vi "MM-TimeSpanText.vi"(4 "Timespan":dbl) -> (1 "TimeSpanText":string)   [LabVIEW 2020]
doc: "Show timespan in text format"
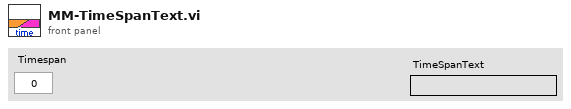
[diagram p1: front panel]
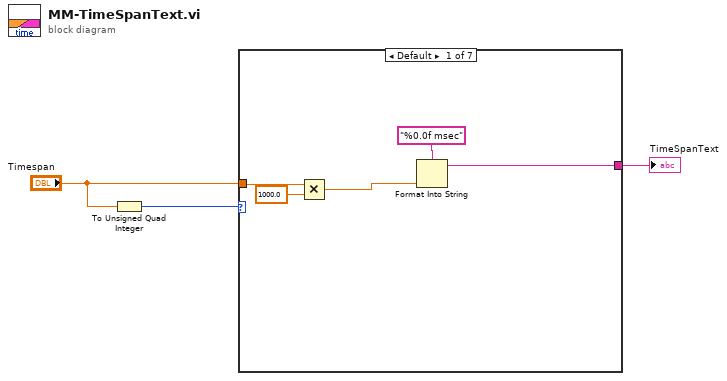
[diagram p0: block diagram]
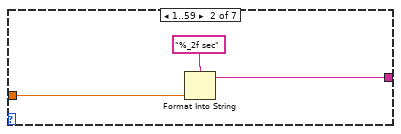
[diagram p2: hidden frame]
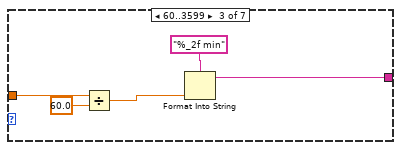
[diagram p3: hidden frame]
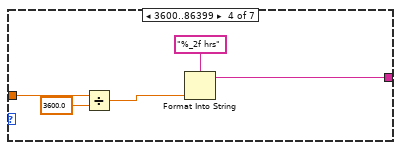
[diagram p4: hidden frame]
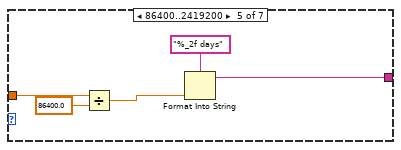
[diagram p5: hidden frame]
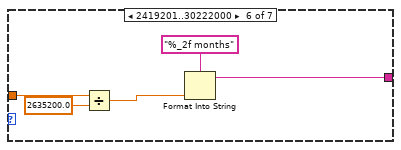
[diagram p6: hidden frame]
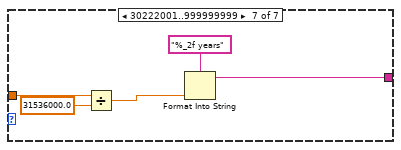
[diagram p7: hidden frame]
diagram:
  n1 = To Unsigned Quad Integer(1:"Timespan") -> (0:w3:u64)
  n2 = case shown="Default" w3 {
    tunnel: "Timespan" -> [w7 w10 w14 w19 w24 w29 w34]
    tunnel: [w4 w9 w15 w20 w25 w30 w35] -> w2
    frame Default {
      n3 = Multiply(x=w7, y=1000.0) -> (x*y=w5:dbl)
      n4 = Format Into String(format string="%0.0f msec", w5) -> (resulting string=w4:string)  [unwired: 2 in, 1 out]
    }
    frame 1..59 {
      n5 = Format Into String(format string="%_2f sec", w10) -> (resulting string=w9:string)  [unwired: 2 in, 1 out]
    }
    frame 60..3599 {
      n6 = Divide(x=w14, y=60.0) -> (x/y=w12:dbl)
      n7 = Format Into String(format string="%_2f min", w12) -> (resulting string=w15:string)  [unwired: 2 in, 1 out]
    }
    frame 3600..86399 {
      n8 = Divide(x=w19, y=3600.0) -> (x/y=w17:dbl)
      n9 = Format Into String(format string="%_2f hrs", w17) -> (resulting string=w20:string)  [unwired: 2 in, 1 out]
    }
    frame 86400..2419200 {
      n10 = Divide(x=w24, y=86400.0) -> (x/y=w22:dbl)
      n11 = Format Into String(format string="%_2f days", w22) -> (resulting string=w25:string)  [unwired: 2 in, 1 out]
    }
    frame 2419201..30222000 {
      n12 = Divide(x=w29, y=2635200.0) -> (x/y=w27:dbl)
      n13 = Format Into String(format string="%_2f months", w27) -> (resulting string=w30:string)  [unwired: 2 in, 1 out]
    }
    frame 30222001..999999999 {
      n14 = Divide(x=w34, y=31536000.0) -> (x/y=w32:dbl)
      n15 = Format Into String(format string="%_2f years", w32) -> (resulting string=w35:string)  [unwired: 2 in, 1 out]
    }
  }
  "TimeSpanText" <- w2
